vi "sub vi - cycle&temp fail v6.vi"(0 "Amps Lo?":bool, 2 "Input Cluster":T1, 3 "SELECT":T2(ring), 4 "Amps Hi?":bool, 5 "Result In":bool) -> (15 "(FAIL) out":cluster{"FAIL LO":dbl, "FAIL HI":dbl}, 16 "(DISP) out":T3, 17 "T-RISE":cluster{"T-RISE (L)":dbl, "T-RISE (N)":dbl}, 18 "Result Out":bool, 19 "file error":errorcluster)   [LabVIEW 2013]
uses:
  program files/Global 1.vi
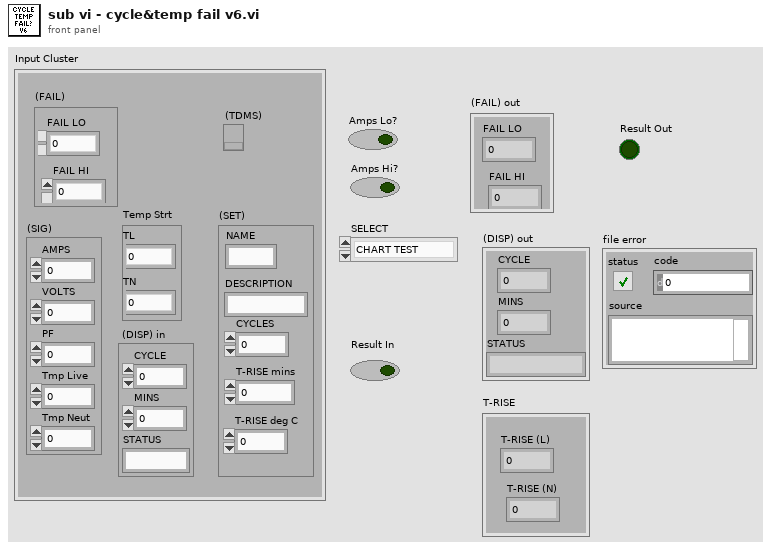
[diagram p1: front panel]
types:
  T1 = cluster{"(FAIL)":cluster{"FAIL LO":dbl, "FAIL HI":dbl}, "(SIG)":cluster{"AMPS":dbl, "VOLTS":dbl, "PF":dbl, "Tmp Live":dbl, "Tmp Neut":dbl}, "Temp Strt":cluster{"TL":dbl, "TN":dbl}, " (DISP) in":cluster{"CYCLE":dbl, "MINS":dbl, "STATUS":string}, "(SET)":cluster{"NAME":string, "DESCRIPTION":string, "CYCLES":dbl, "T-RISE mins":dbl, "T-RISE deg C":dbl}, "(TDMS)":refnum<k34>}
  T2 = enum32{"CHART TEST", "CYCLE TEST", "T-RISE TEST"}
  T3 = cluster{"CYCLE":dbl, "MINS":dbl, "STATUS":string}
  T4 = cluster{"AMPS":dbl, "VOLTS":dbl, "PF":dbl, "Tmp Live":dbl, "Tmp Neut":dbl}
  T5 = cluster{"NAME":string, "DESCRIPTION":string, "CYCLES":dbl, "T-RISE mins":dbl, "T-RISE deg C":dbl}
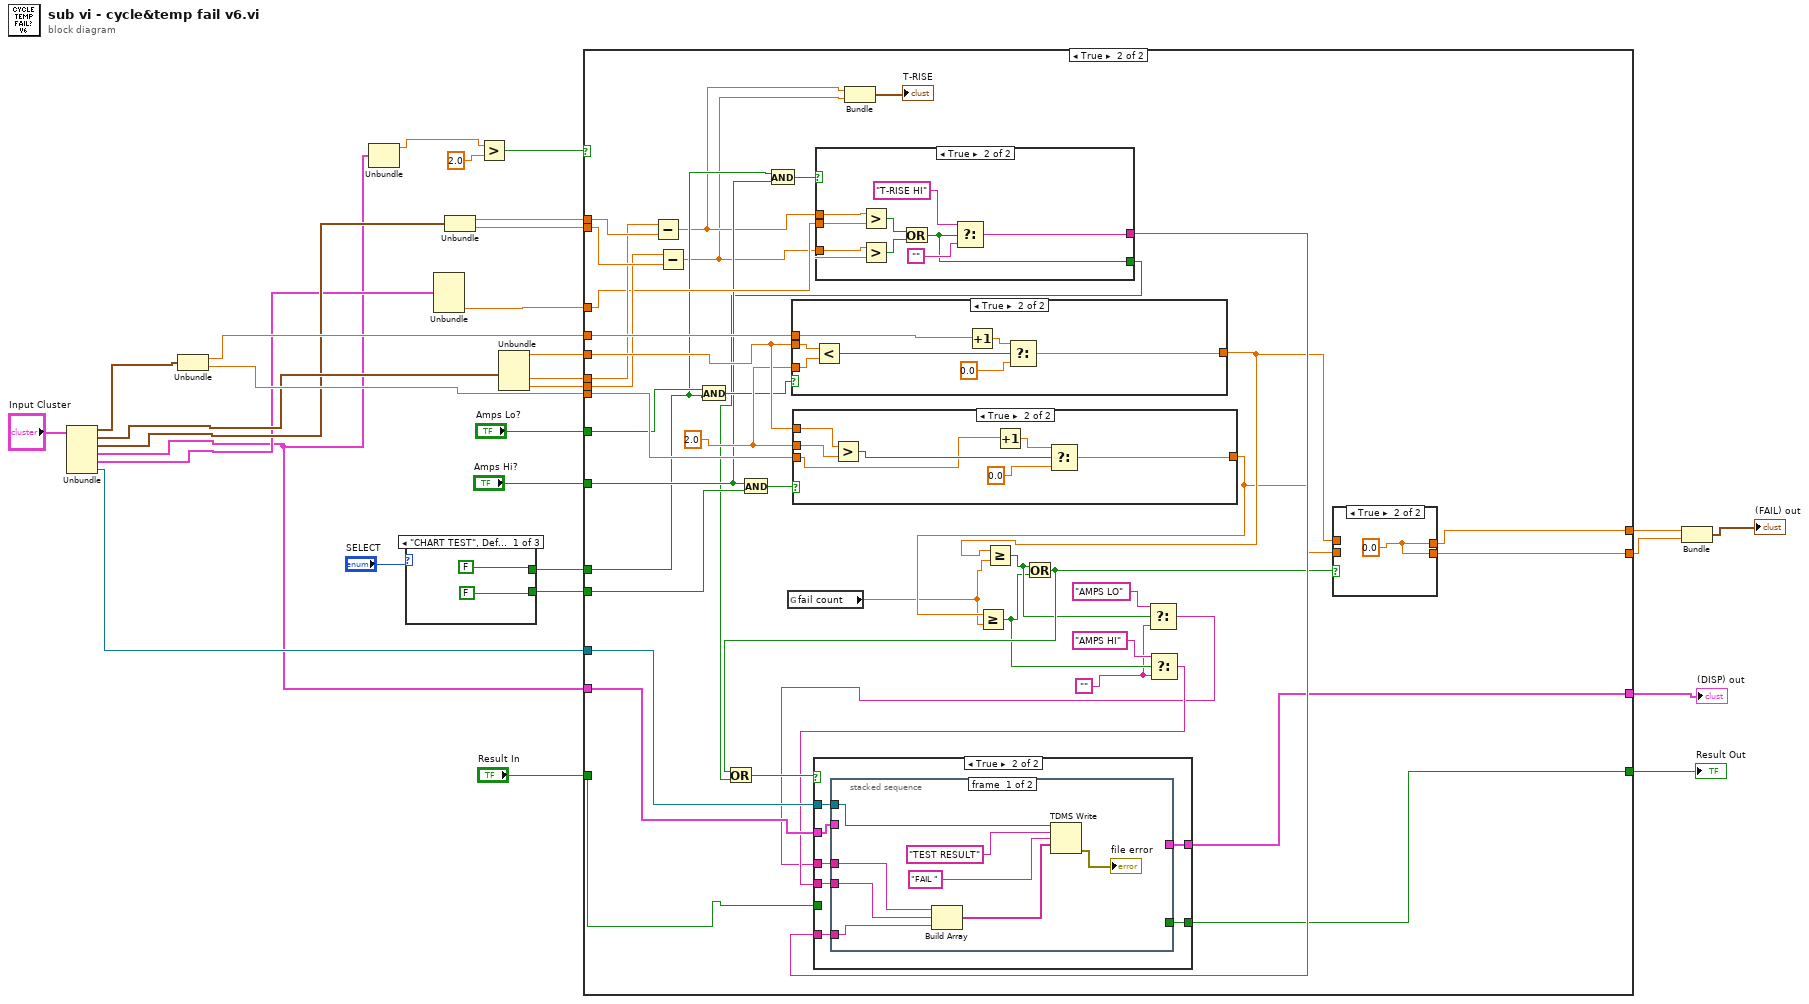
[diagram p0: block diagram]
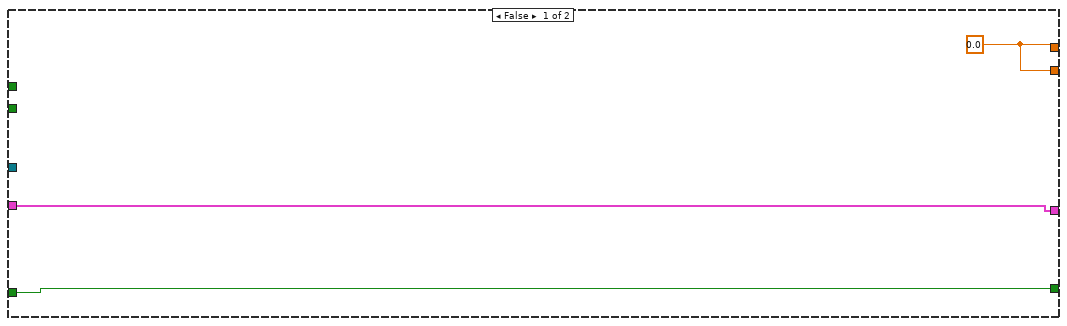
[diagram p2: hidden frame]
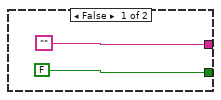
[diagram p4: hidden frame]
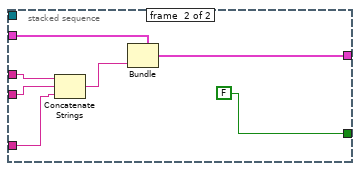
[diagram p6: hidden frame]
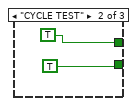
[diagram p9: hidden frame]
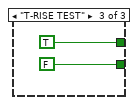
[diagram p10: hidden frame]
diagram:
  n1 = Unbundle("Input Cluster") -> ("(FAIL)"=w15:cluster{"FAIL LO":dbl, "FAIL HI":dbl}, "(SIG)"=w12:T4, "Temp Strt"=w11:cluster{"TL":dbl, "TN":dbl}, "(DISP) in"=w2:T3, "(SET)"=w10:T5, "(TDMS)"=w9:refnum<k34>)
  n2 = Unbundle(w15) -> ("FAIL LO"=w14:dbl, "FAIL HI"=w13:dbl)
  n3 = Unbundle(w2) -> ("CYCLE"=w1:dbl)  [unwired: 2 out]
  n4 = case shown="\"CHART TEST\", Default" "SELECT" {
    tunnel: [FALSE TRUE TRUE] -> w19
    tunnel: [FALSE TRUE FALSE] -> w22
    frame "CHART TEST", Default {
    }
    frame "CYCLE TEST" {
    }
    frame "T-RISE TEST" {
    }
  }
  n5 = Unbundle(w10) -> ("T-RISE deg C"=w23:dbl)  [unwired: 4 out]
  n6 = Unbundle(w11) -> ("TL"=w27:dbl, "TN"=w26:dbl)
  n7 = Greater?(x=w1, y=2.0) -> (0:w17:bool)
  n8 = Unbundle(w12) -> ("AMPS"=w28:dbl, "Tmp Live"=w25:dbl, "Tmp Neut"=w24:dbl)  [unwired: 2 out]
  n9 = case shown="True" w17 {
    tunnel: w28 -> [_ w78]
    tunnel: w14 -> [_ w76]
    tunnel: w13 -> [_ w75]
    tunnel: w9 -> [_ w74]
    tunnel: w2 -> [w37 w73]
    tunnel: w27 -> [_ w72]
    tunnel: w26 -> [_ w71]
    tunnel: w25 -> [_ w70]
    tunnel: w24 -> [_ w69]
    tunnel: w23 -> [_ w68]
    tunnel: w22 -> [_ w65]
    tunnel: "Amps Lo?" -> [_ w63]
    tunnel: "Amps Hi?" -> [_ w61]
    tunnel: w19 -> [_ w60]
    tunnel: [w38 w57] -> w7
    tunnel: [w38 w56] -> w6
    tunnel: [w37 w55] -> w5
    tunnel: [w36 w54] -> w4
    tunnel: "Result In" -> [w36 w53]
    frame False {
      w38 = 0.0
    }
    frame True {
      w45 = ""
      w77 = 2.0
      n10 = Subtract(x=w70, y=w72) -> (x-y=w42:dbl)
      n11 = Subtract(x=w69, y=w71) -> (x-y=w41:dbl)
      n12 = And(x=w63, y=w60) -> (x .and. y?=w64:bool)
      n13 = And(x=w61, y=w65) -> (x .and. y?=w66:bool)
      n14 = And(x=w60, y=w61) -> (x .and. y?=w62:bool)
      n15 = global read "Global 1.vi" "fail count"() -> (w39:dbl)
      n16 = case shown="True" w64 {
        tunnel: w78 -> [_ w132]
        tunnel: w77 -> [_ w131]
        tunnel: w76 -> [w125 w127]
        tunnel: [w125 w126] -> w59
        frame False {
        }
        frame True {
          n17 = Less?(x=w132, y=w131) -> (x < y?=w130:bool)
          n18 = Increment(x=w127) -> (x+1=w129:dbl)
          n19 = Select(t=w129, s=w130, f=0.0) -> (s? t:f=w126:dbl)
        }
      }
      n20 = case shown="True" w66 {
        tunnel: w78 -> [_ w124]
        tunnel: w77 -> [_ w123]
        tunnel: [w117 w119] -> w58
        tunnel: w75 -> [w117 w118]
        frame False {
        }
        frame True {
          n21 = Greater?(x=w124, y=w123) -> (0:w122:bool)
          n22 = Increment(x=w118) -> (x+1=w121:dbl)
          n23 = Select(t=w121, s=w122, f=0.0) -> (s? t:f=w119:dbl)
        }
      }
      n24 = case shown="True" w62 {
        tunnel: w68 -> [_ w92]
        tunnel: w42 -> [_ w85]
        tunnel: w41 -> [_ w84]
        tunnel: ["" w87] -> w67
        tunnel: [FALSE w86] -> w51
        frame False {
        }
        frame True {
          n25 = Greater?(x=w85, y=w92) -> (0:w90:bool)
          n26 = Greater?(x=w84, y=w92) -> (0:w91:bool)
          n27 = Or(x=w90, y=w91) -> (x .or. y?=w86:bool)
          n28 = Select(t="T-RISE HI", s=w86, f="") -> (s? t:f=w87:string)
        }
      }
      n29 = Bundle(w42, w41) -> (→"T-RISE":cluster{dbl, dbl})  [unwired: 1 in]
      n30 = Greater Or Equal?(x=w58, y=w39) -> (x >= y?=w48:bool)
      n31 = Greater Or Equal?(x=w59, y=w39) -> (x >= y?=w49:bool)
      n32 = Or(x=w49, y=w48) -> (x .or. y?=w52:bool)
      n33 = Or(x=w52, y=w51) -> (x .or. y?=w50:bool)
      n34 = Select(t="AMPS LO", s=w49, f=w45) -> (s? t:f=w43:string)
      n35 = Select(t="AMPS HI", s=w48, f=w45) -> (s? t:f=w44:string)
      n36 = case shown="True" w50 {
        tunnel: w43 -> [_ w101]
        tunnel: w44 -> [_ w100]
        tunnel: w73 -> [w94 w99]
        tunnel: w74 -> [_ w98]
        tunnel: w67 -> [_ w97]
        tunnel: [w94 w96] -> w55
        tunnel: [w93 w95] -> w54
        tunnel: w53 -> [w93 _]
        frame False {
        }
        frame True {
          n37 = stacked-sequence {
            tunnel: w101 -> [w102 w116]
            tunnel: w100 -> [w103 w115]
            tunnel: w99 -> [_ w113]
            tunnel: w98 -> [w105 _]
            tunnel: w97 -> [w104 w112]
            tunnel: [_ w111] -> w96
            tunnel: [_ FALSE] -> w95
            frame #0 {
              n38 = Build Array(w102, w103, w104) -> (w108:string[])
              n39 = TDMS Write(0:w105, 5:"TEST RESULT", 7:"FAIL ", 9:w108) -> (15:→"file error":errorcluster)  [unwired: 2 in, 3 out]
            }
            frame #1 {
              n40 = Concatenate Strings(w116, w115, w112) -> (w114:string)
              n41 = Bundle(cluster=w113, "STATUS"=w114) -> (w111:T3)  [unwired: 2 in]
            }
          }
        }
      }
      n42 = case shown="True" w52 {
        tunnel: w59 -> [w80 _]
        tunnel: w58 -> [w79 _]
        tunnel: [w80 w81] -> w57
        tunnel: [w79 w81] -> w56
        frame False {
        }
        frame True {
          w81 = 0.0
        }
      }
    }
  }
  "(DISP) out" <- w5
  "Result Out" <- w4
  n43 = Bundle("FAIL LO"=w7, "FAIL HI"=w6) -> (→"(FAIL) out":cluster{"FAIL LO":dbl, "FAIL HI":dbl})  [unwired: 1 in]
